vi "5.11-OCU TCP Send Client.vi"() -> ()   [LabVIEW 2010]
doc: "Displays data sent via TCP from Data Server.vi. Once a TCP connection is open, the VI reads 4 bytes to determine the amount of data being sent. It then reads and charts that many bytes. If an error occurs or the stop button is pressed, it sends a \"Q\" to the Data Sender to notify it to quit.\n\n<B>Note:</B> Requires the Data Server.vi located in the same library as this VI."
uses:
  7-OCU/7.0-Global.vi
  5.0-Global.vi
panel:
  in  "Address":string="10.10.10.2"
  in  "Port":u16=53483 min=1025 step=1
  # "Instructions:\n1. Open the Data Server.vi located in the same library.\n2. Follow the instructions on it's front panel.\n\nNote: This VI is built to work with the Data Server.vi."
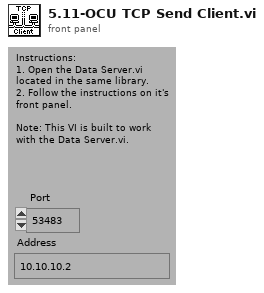
[diagram p1: front panel]
types:
  T1 = typedef "6.1-Act.ctl" = cluster{"6.1-Saitek Controller":T2, "Joystick Mode":bool, "Shutdown":bool, "Reset":bool, "Begin":bool}
  T2 = typedef "6.1-UDP Saitek.ctl" = cluster{"Stop":bool, "Setpoint":bool, "Run":bool, "Restart":bool, "Shutdown":bool, "Joystick\nMode 1":bool, "Joystick\nMode 2":bool, "Joystick \nMode 3":bool, "Joystick Mode 4":bool, "10":bool, "11":bool, "Pitch":sgl, "Roll":sgl, "Yaw":sgl, "Left":sgl, "Right":sgl}
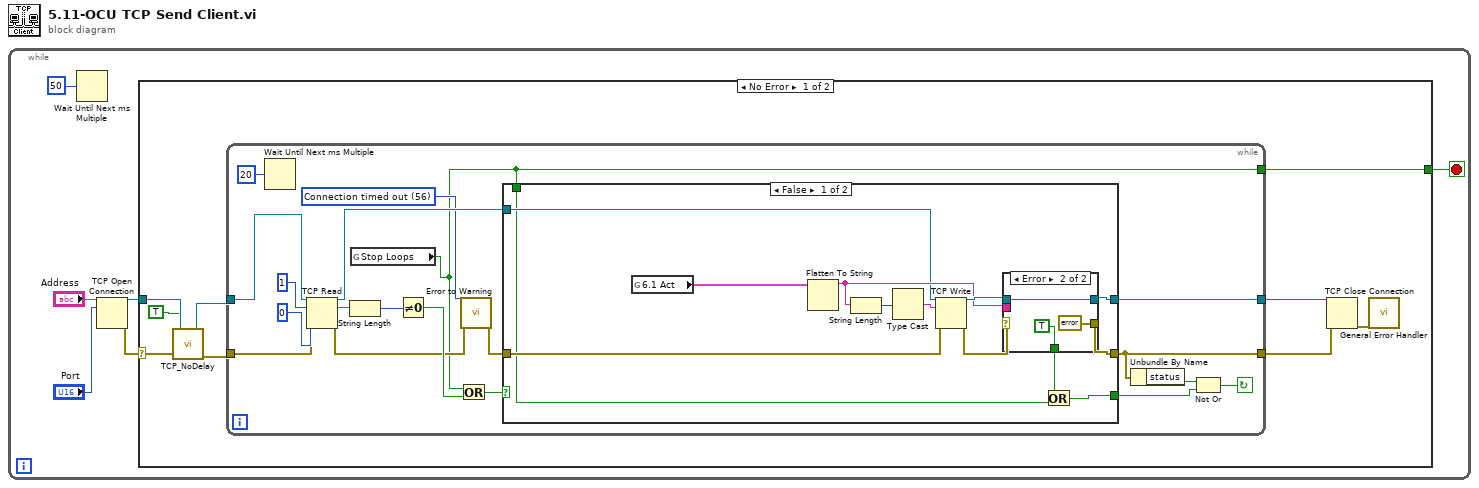
[diagram p0: block diagram]
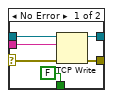
[diagram p2: hidden frame]
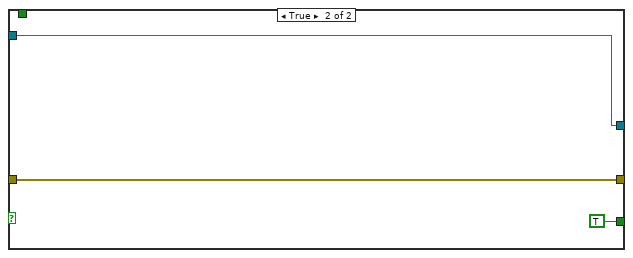
[diagram p3: hidden frame]
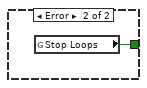
[diagram p4: hidden frame]
diagram:
  n1 = while {
    stop <- w1 stop-if-true
    n2 = Wait Until Next ms Multiple(millisecond multiple=u32 50) -> ()  [unwired: 1 out]
    n3 = TCP Open Connection(address="Address", remote port or service name="Port") -> (connection ID=w4:refnum<k5>, error out=w3:errorcluster)  [unwired: 1 in, 2 out]
    n4 = case shown="No Error" w3 {
      selector: w3 -> [w8 _]
      tunnel: w4 -> [w11 _]
      tunnel: [w14 w60] -> w1
      frame No Error {
        n5 = call "TCP_NoDelay.vi"("error in (no error)"=w8, "TCP_NODELAY (true)"=TRUE, "connID"=w11) -> ("error out"=w9:errorcluster, "connID 2"=w10:refnum<k5>)  [unwired: 3 in]
        n6 = while {
          tunnel: [w16] -> w14
          tunnel: [w26] -> w12
          tunnel: w10 -> [w19]
          tunnel: [w21] -> w13
          tunnel: w9 -> [w20]
          stop <- w34 continue-if-true
          w24 = 56 items=["No Error", "Argument Error", "Memory Full", "Out of Zone", "End of File", "File Already Open", "Generic File IO Error", "File Not Found", "File Permission Error", "Disk Full", "Duplicate Path", "Too Many Files Open", "Not Enabled", "Resource File Not Found", "Cannot Add Resource", "Resource Not Found", "Image Not Found", "Image Memory Error", "Pen Does Not Exist", "Config Bad Type", "Config Token Not Found", "Config Parse Error", "Config Memory Error", "Bad External Code Format", "Bad External Code Offset", "External Code Not Present", "Null Window", "Destroy Window Mixup", "Null Menu", "Print Aborted", "Bad Print Record", "Print Driver Error", "Windows Error During Print", "Memory Error During Print", "Print Dialog Error", "Generic Print Error", "Invalid Device Refnum", "Device Not Found", "Device Parameter Error", "Device Unit Error", "Can't Open Device", "Device Call Aborted", "Generic Error", "Cancelled By User", "Object ID Too Low", "Object ID Too High", "Object Not In Heap", "Unknown Heap", "Bad DefProc ID", "DefProc Not In Table", "Message Out Of Range", "Null Method", "Unknown Message", "Manager Call Not Supported", "Bad address", "Connection In progress", "Connection timed out", "Connection is already in progress", "Network attribute not supported", "Network error", "Address in use", "System out of memory", "Connection aborted", "Connection refused", "Connection is not connected", "Connection is already connected", "Connection closed", "Initialize error (interapplication manager)", "Bad occurrence", "Wait on unbound occurrence handler", "Occurrence queue overflow", "Bad path", "Semaphore not signaled", "Unrecognized type (interapplication manager)"] ("1st Error to Convert")
          n7 = Wait Until Next ms Multiple(millisecond multiple=u32 20) -> ()  [unwired: 1 out]
          n8 = TCP Read(connection ID=w19, bytes to read=1, error in (no error)=w20, 9:0) -> (connection ID out=w30:refnum<k5>, data out=w31:string, error out=w23:errorcluster)  [unwired: 1 in]
          n9 = String Length(string=w31) -> (length=w29:i32)
          n10 = global read "7.0-Global.vi" "Stop Loops"() -> (w16:bool)
          n11 = Not Equal To 0?(x=w29) -> (x != 0?=w28:bool)
          n12 = Or(x=w16, y=w28) -> (x .or. y?=w27:bool)
          n13 = call <vilib>:"Error to Warning.vi"("1st Error to Convert"=w24, "error in"=w23) -> ("warning out"=w22:errorcluster)  [unwired: 13 in]
          n14 = case shown="False" w27 {
            tunnel: w22 -> [w44 w57]
            tunnel: w30 -> [w40 w58]
            tunnel: [w43 w58] -> w21
            tunnel: [w42 w57] -> w26
            tunnel: [w38 TRUE] -> w17
            tunnel: w16 -> [w39 _]
            frame False {
              n15 = global read "7.0-Global.vi" "6.1 Act"() -> (w35:T1)
              n16 = Flatten To String(anything=w35) -> (data string=w41:string)  [unwired: 3 in, 2 out]
              n17 = String Length(string=w41) -> (length=w46:i32)
              n18 = Type Cast(x=w46) -> (*(type *) &x=w47:string)  [unwired: 1 in]
              n19 = TCP Write(connection ID=w40, data in=w47, error in (no error)=w44) -> (connection ID out=w45:refnum<k5>, error out=w36:errorcluster)  [unwired: 1 in, 1 out]
              n20 = case shown="Error" w36 {
                selector: w36 -> [w50 _]
                tunnel: w45 -> [w53 w55]
                tunnel: [w48 w55] -> w43
                tunnel: [w49 errorcluster {"status"=FALSE, "code"=0, "source"=""} ("error out")] -> w42
                tunnel: w41 -> [w52 _]
                tunnel: [FALSE ("x") TRUE ("x")] -> w37
                frame No Error {
                  n21 = TCP Write(connection ID=w53, data in=w52, error in (no error)=w50) -> (connection ID out=w48:refnum<k5>, error out=w49:errorcluster)  [unwired: 1 in, 1 out]
                }
                frame Error {
                }
              }
              n22 = Or(x=w37, y=w39) -> (x .or. y?=w38:bool)
            }
            frame True {
            }
          }
          n23 = Unbundle By Name(w26) -> ("status"=w25:bool)
          n24 = Not Or(1:w17, 2:w25) -> (0:w34:bool)
        }
        n25 = TCP Close Connection(connection ID=w13, error in (no error)=w12) -> (error out=w15:errorcluster)  [unwired: 2 out]
        n26 = call <vilib>:"General Error Handler.vi"("error in (no error)"=w15) -> ()  [unwired: 1 in, 14 out]
      }
      frame Error {
        n27 = global read "5.0-Global.vi" "Stop Loops"() -> (w60:bool)
      }
    }
  }
